vi "快关最值.vi"(4 "计算参数 in":T2, 5 "输入参数 in":T1, 7 "Array in":dbl[](array[numeric])) -> (0 "计算参数 out":T2, 1 "输入参数 out":T1, 3 "Array out":dbl[](array[numeric]))   [LabVIEW 2013]
doc: "将数组首部100个元素的平均值作为100%时的电流值，将数组尾部100个元素的平均值作为0%时的电流值"
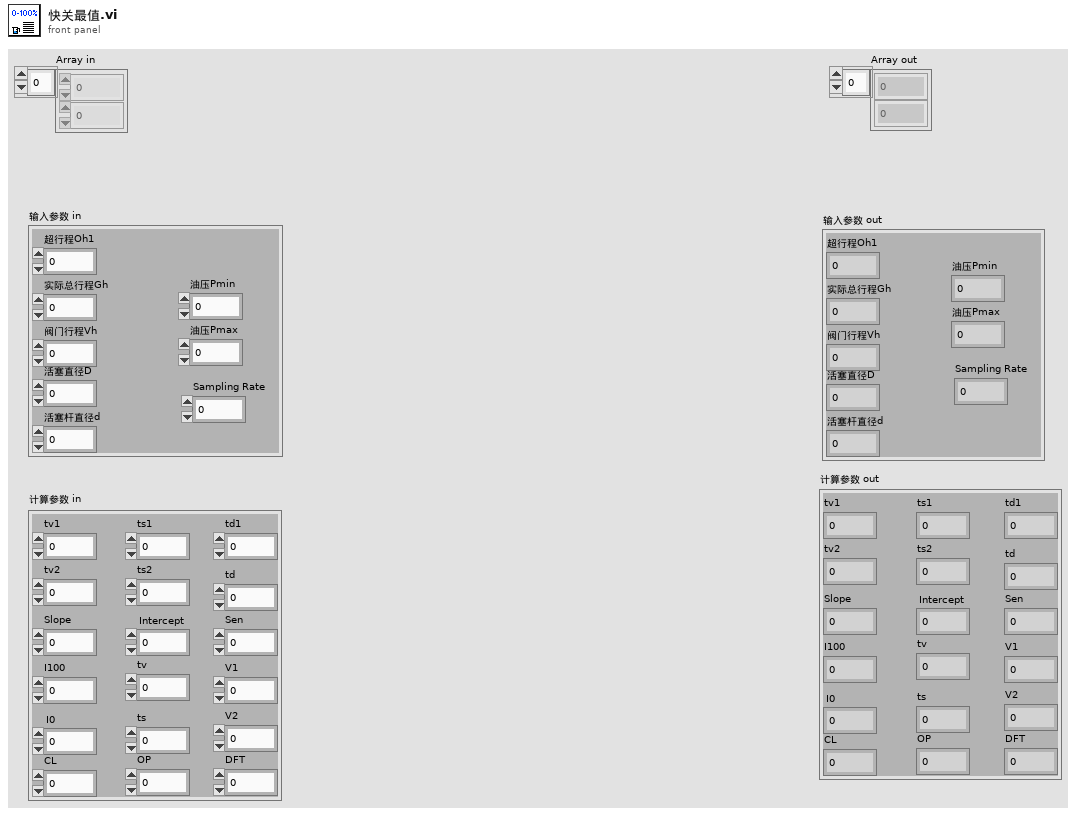
[diagram p1: front panel]
types:
  T1 = cluster{"超行程Oh1":dbl, "实际总行程Gh":dbl, "阀门行程Vh":dbl, "活塞直径D":dbl, "活塞杆直径d":dbl, "油压Pmin":dbl, "油压Pmax":dbl, "Sampling Rate":dbl}
  T2 = cluster{"tv1":dbl, "tv2":dbl, "tv":dbl, "ts1":dbl, "ts2":dbl, "ts":dbl, "td1":dbl, "td":dbl, "Slope":dbl, "Intercept":dbl, "I100":dbl, "I0":dbl, "Sen":dbl, "V1":dbl, "V2":dbl, "CL":dbl, "OP":dbl, "DFT":dbl}
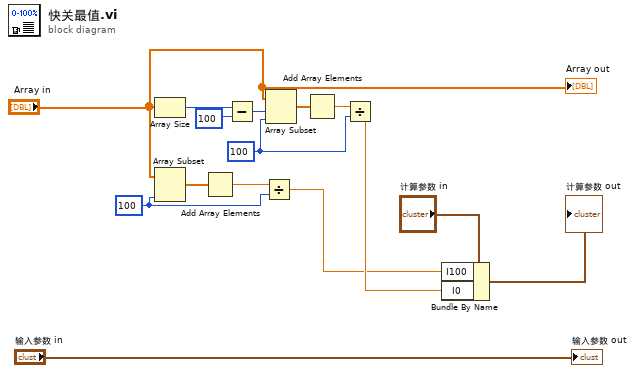
[diagram p0: block diagram]
diagram:
  w11 = 100 ("长度")
  w10 = 100 ("长度")
  n1 = Array Size(array="Array in") -> (size(s)=w15:i32)
  n2 = Array Subset(array="Array in", length=w10) -> (w8:dbl[])  [unwired: 1 in]
  n3 = Add Array Elements(numeric array=w8) -> (sum=w9:dbl)
  n4 = Subtract(x=w15, y=100) -> (x-y=w13:i32)
  n5 = Divide(x=w9, y=w10) -> (x/y=w3:dbl)
  n6 = Array Subset(array="Array in", index=w13, length=w11) -> (w6:dbl[])
  n7 = Add Array Elements(numeric array=w6) -> (sum=w12:dbl)
  n8 = Divide(x=w12, y=w11) -> (x/y=w4:dbl)
  n9 = Bundle By Name(cluster="计算参数 in", "I100"=w3, "I0"=w4) -> (→"计算参数 out":T2)
  "Array out" <- "Array in"
  "输入参数 out" <- "输入参数 in"
